vi "Write.2DLIF.vi"(8 "Mono":T2, 9 "DyeLaser":T3, 10 "Camera":T1={"Gate.Delay"=0, "Delay.Step"=0, "Gate.Duration"=150000, "#Accum"=10, "SetpointTemp"=-30, "Last Temp"=6, "Current Temp"=4}, 11 "Data":cluster{"CCD":i32[], "2D LIF plot":i32[][]}) -> (3 "last saved file":path)   [LabVIEW 2022 SP3]
uses:
  <vilib>/Utility/file.llb/Write Delimited Spreadsheet (I64).vi
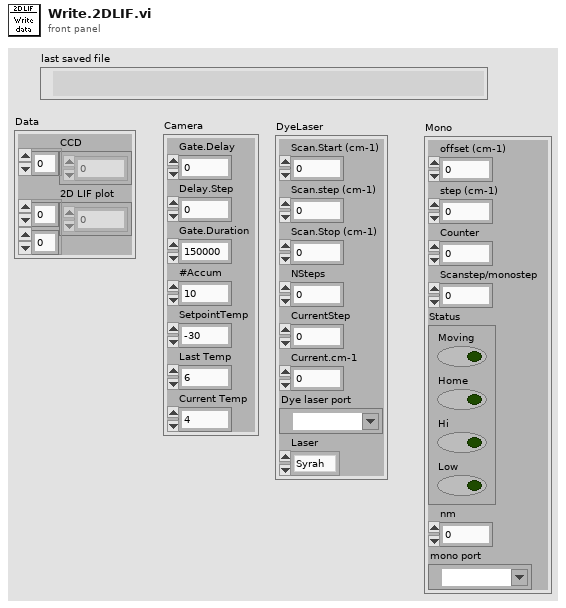
[diagram p1: front panel]
types:
  T1 = cluster{"Gate.Delay":u64, "Delay.Step":u64, "Gate.Duration":u64, "#Accum":i32, "SetpointTemp":i32, "Last Temp":i32, "Current Temp":i32}
  T2 = cluster{"offset (cm-1)":dbl, "step (cm-1)":dbl, "Counter":dbl, "Scanstep/monostep":i32, "Status":cluster{"Moving":bool, "Home":bool, "Hi":bool, "Low":bool}, "nm":dbl, "mono port":refnum<visa-resource-name>}
  T3 = cluster{"Scan.Start (cm-1)":dbl, "Scan.Stop (cm-1)":dbl, "Scan.step (cm-1)":dbl, "Dye laser port":refnum<visa-resource-name>, "Laser":enum16{"Syrah", "Hyperdye"}, "NSteps":i32, "CurrentStep":i32, "Current.cm-1":dbl}
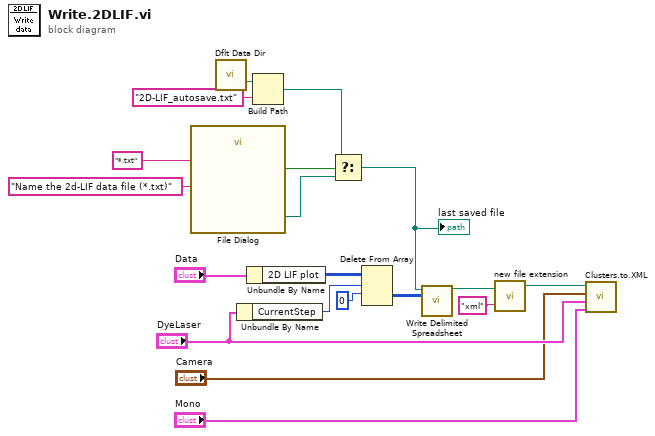
[diagram p0: block diagram]
diagram:
  n1 = call "File Dialog"("prompt"="Name the 2d-LIF data file (*.txt)", "pattern (all files)"="*.txt" ("default name")) -> ("selected path"=w2:path, "cancelled"=w4:bool)  [unwired: 10 in, 2 out]
  n2 = call <vilib>:"Dflt Data Dir.vi"() -> ("App:Default Data Directory"=w6:path)
  n3 = Unbundle By Name("DyeLaser") -> ("CurrentStep"=w11:i32)
  n4 = Unbundle By Name("Data") -> ("2D LIF plot"=w10:i32[][])
  n5 = Build Path(base path=w6, name or relative path="2D-LIF_autosave.txt") -> (appended path=w3:path)
  n6 = Select(t=w3, s=w4, f=w2) -> (s? t:f=w1:path)
  "last saved file" <- w1
  n7 = Delete From Array(array=w10, length=w11, index (row)=0) -> (deleted portion=w14:i32[][])  [unwired: 1 in, 1 out]
  n8 = call-poly <vilib>:"Write Delimited Spreadsheet.vi"("file path (dialog if empty)"=w1, "2D data"=w14) -> ("new file path (Not A Path if cancelled)"=w15:path)  [unwired: 12 in, 1 out]
  n9 = call "new file extension.vi"("new extension"="xml", "input path"=w15) -> ("output path&filename"=w17:path)
  n10 = call "Clusters.to.XML.vi"("Mono"="Mono", "DyeLaser"="DyeLaser", "Camera"="Camera", "XML File Path"=w17) -> ()  [unwired: 8 in]
